vi "Apply Graph Property.vi"(6 "Display State Change Class":T2, 8 "error in (no error)":errorcluster, 9 "Max Range":T1, 10 "XY Graph Property Cluster":T3, 11 "XY Graph":refnum<vi>) -> (0 "error out":errorcluster, 3 "XY Graph":refnum<vi>)   [LabVIEW 2020, in "XY Plot Matrix.lvclass"]
uses:
  <vilib>/Math Plots/2D Math Plots/XY Plot Matrix/XY Plot Matrix/XY Plot Matrix.lvclass
  <vilib>/Math Plots/2D Math Plots/2D Plot/2D Plot/Typedef/Property Cluster.ctl
  <vilib>/Math Plots/2D Math Plots/2D Plot/2D Plot/Typedef/Graph General Property.ctl
  <vilib>/Math Plots/2D Math Plots/2D Plot/2D Plot/Typedef/Scale Array.ctl
  <vilib>/Math Plots/2D Math Plots/2D Plot/2D Plot/Typedef/Scale Cluster.ctl
  <vilib>/Utility/miscctls.llb/LVOffsetAndMultiplierTypeDef.ctl
  <vilib>/Math Plots/2D Math Plots/2D Plot/2D Plot/Typedef/Cursor Property.ctl
  <vilib>/Utility/miscctls.llb/LVCursorListTypeDef.ctl
  <vilib>/Utility/miscctls.llb/LVAnnotationListTypeDef.ctl
  <vilib>/Math Plots/2D Math Plots/2D Plot/Action String/2DMathPlot State Class.ctl
  <vilib>/Math Plots/2D Math Plots/2D Plot/2D Plot/Typedef/Range Cluster.ctl
  <vilib>/Math Plots/2D Math Plots/2D Plot/2D Plot/2D Plot.lvclass
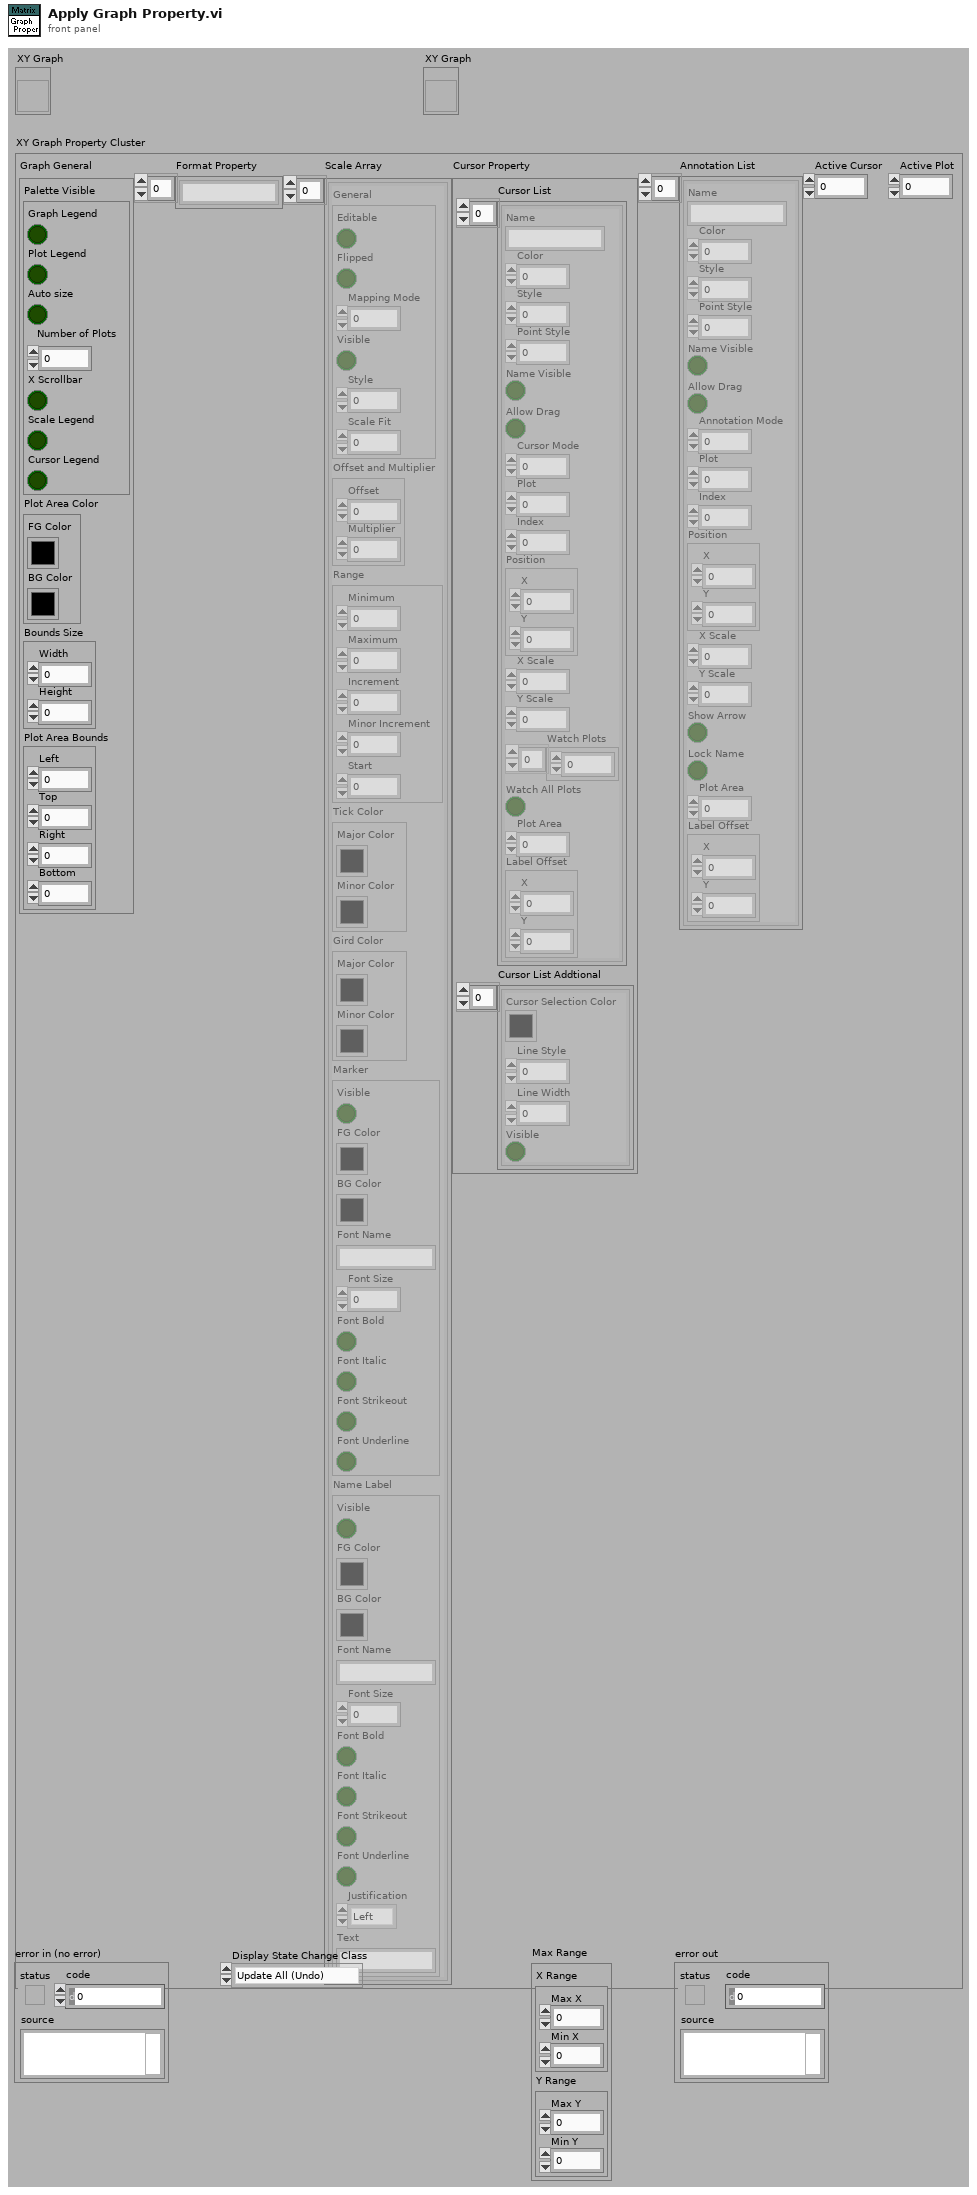
[diagram p1: front panel]
types:
  T1 = typedef "2D Plot.lvclass/Range Cluster.ctl" = cluster{"X Range":cluster{"Max X":dbl, "Min X":dbl}, "Y Range":cluster{"Max Y":dbl, "Min Y":dbl}}
  T2 = typedef "2DMathPlot State Class.ctl" = enum16{"Update All (Undo)", "Update General", "Update Appearance", "Update Format", "Update Scale", "Update Marker", "Update Cursor", "None"}
  T3 = typedef "2D Plot.lvclass/Property Cluster.ctl" = cluster{"Graph General":T4, "Format Property":string[], "Scale Array":T5, "Cursor Property":T8, "Annotation List":T10, "Active Cursor":i32, "Active Plot":i32}
  T4 = typedef "2D Plot.lvclass/Graph General Property.ctl" = cluster{"Palette Visible":cluster{"Graph Legend":bool, "Plot Legend":bool, "Auto size":bool, "Number of Plots":u32, "X Scrollbar":bool, "Scale Legend":bool, "Cursor Legend":bool}, "Plot Area Color":cluster{"FG Color":u32, "BG Color":u32}, "Bounds Size":cluster{"Width":u32, "Height":u32}, "Plot Area Bounds":cluster{"Left":i16, "Top":i16, "Right":i16, "Bottom":i16}}
  T5 = typedef "2D Plot.lvclass/Scale Array.ctl" = T6[]
  T6 = typedef "2D Plot.lvclass/Scale Cluster.ctl" = cluster{"General":cluster{"Editable":bool, "Flipped":bool, "Mapping Mode":u8, "Visible":bool, "Style":u8, "Scale Fit":u8}, "Offset and Multiplier":T7, "Range":cluster{"Minimum":dbl, "Maximum":dbl, "Increment":dbl, "Minor Increment":dbl, "Start":dbl}, "Tick Color":cluster{"Major Color":u32, "Minor Color":u32}, "Gird Color":cluster{"Major Color":u32, "Minor Color":u32}, "Marker":cluster{"Visible":bool, "FG Color":u32, "BG Color":u32, "Font Name":string, "Font Size":u32, "Font Bold":bool, "Font Italic":bool, "Font Strikeout":bool, "Font Underline":bool}, "Name Label":cluster{"Visible":bool, "FG Color":u32, "BG Color":u32, "Font Name":string, "Font Size":u32, "Font Bold":bool, "Font Italic":bool, "Font Strikeout":bool, "Font Underline":bool, "Justification":enum16{"Left", "Center", "Right"}, "Text":string}}
  T7 = typedef "LVOffsetAndMultiplierTypeDef.ctl" = cluster{"Offset":dbl, "Multiplier":dbl}
  T8 = typedef "2D Plot.lvclass/Cursor Property.ctl" = cluster{"Cursor List":T9, "Cursor List Addtional":cluster{"Cursor Selection Color":u32, "Line Style":u8, "Line Width":u8, "Visible":bool}[]}
  T9 = typedef "LVCursorListTypeDef.ctl" = cluster{"Name":string, "Color":u32, "Style":u8, "Point Style":u8, "Name Visible":bool, "Allow Drag":bool, "Cursor Mode":u32, "Plot":i32, "Index":i32, "Position":cluster{"X":dbl, "Y":dbl}, "X Scale":u32, "Y Scale":u32, "Watch Plots":i32[], "Watch All Plots":bool, "Plot Area":i32, "Label Offset":cluster{"X":dbl, "Y":dbl}}[]
  T10 = typedef "LVAnnotationListTypeDef.ctl" = cluster{"Name":string, "Color":u32, "Style":u8, "Point Style":u8, "Name Visible":bool, "Allow Drag":bool, "Annotation Mode":u32, "Plot":i32, "Index":i32, "Position":cluster{"X":dbl, "Y":dbl}, "X Scale":u32, "Y Scale":u32, "Show Arrow":bool, "Lock Name":bool, "Plot Area":i32, "Label Offset":cluster{"X":dbl, "Y":dbl}}[]
  T11 = cluster{"Graph Legend":bool, "Plot Legend":bool, "Auto size":bool, "Number of Plots":u32, "X Scrollbar":bool, "Scale Legend":bool, "Cursor Legend":bool}
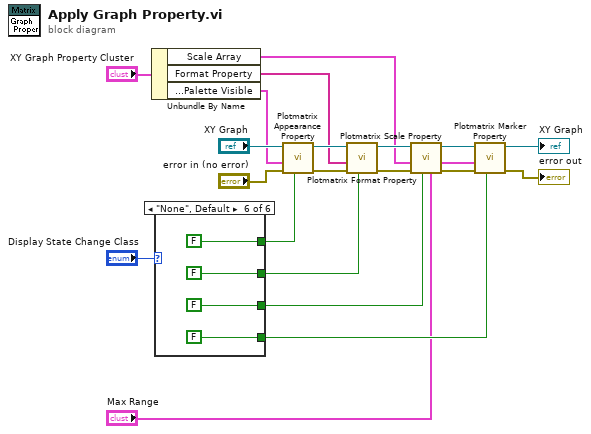
[diagram p0: block diagram]
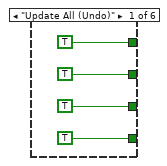
[diagram p2: hidden frame]
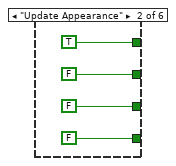
[diagram p3: hidden frame]
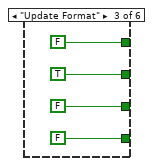
[diagram p4: hidden frame]
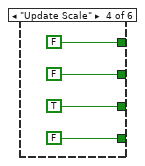
[diagram p5: hidden frame]
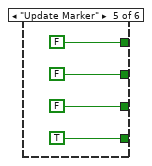
[diagram p6: hidden frame]
diagram:
  n1 = Unbundle By Name("XY Graph Property Cluster") -> ("Scale Array"=w12:T5, "Format Property"=w7:string[], "Graph General.Palette Visible"=w13:T11)
  n2 = case shown="\"None\", Default" "Display State Change Class" {
    tunnel: [TRUE ("Update?") TRUE ("Update?") FALSE ("Update?") FALSE ("Update?") FALSE ("Update?") FALSE ("Update?")] -> w5
    tunnel: [TRUE ("Update?") FALSE ("Update?") TRUE ("Update?") FALSE ("Update?") FALSE ("Update?") FALSE ("Update?")] -> w4
    tunnel: [TRUE ("Update?") FALSE ("Update?") FALSE ("Update?") TRUE ("Update?") FALSE ("Update?") FALSE ("Update?")] -> w3
    tunnel: [TRUE ("Update?") FALSE ("Update?") FALSE ("Update?") FALSE ("Update?") TRUE ("Update?") FALSE ("Update?")] -> w2
    frame "Update All (Undo)" {
    }
    frame "Update Appearance" {
    }
    frame "Update Format" {
    }
    frame "Update Scale" {
    }
    frame "Update Marker" {
    }
    frame "None", Default {
    }
  }
  n3 = call <vilib>:"Plotmatrix Appearance Property.vi"("Update?"=w5, "error in (no error)"="error in (no error)", "Palette Visible"=w13, "Single XY Plot In"="XY Graph") -> ("error out"=w8:errorcluster, "Single XY Plot Out"=w19:refnum<vi>)  [unwired: 1 in, 5 out]
  n4 = call <vilib>:"Plotmatrix Format Property.vi"("Update?"=w4, "error in (no error)"=w8, "Format Property"=w7, "Single XY Plot In"=w19) -> ("error out"=w9:errorcluster, "Single XY Plot Out"=w18:refnum<vi>)  [unwired: 6 out]
  n5 = call <vilib>:"Plotmatrix Scale Property.vi"("Max Range"="Max Range", "Update?"=w3, "error in (no error)"=w9, "Scale Array In"=w12, "Single XY Plot In"=w18) -> ("error out"=w10:errorcluster, "Scale Array Out"=w11:T5, "Single XY Plot Out"=w17:refnum<vi>)  [unwired: 4 out]
  n6 = call <vilib>:"Plotmatrix Marker Property.vi"("Update?"=w2, "error in (no error)"=w10, "Scale Array In"=w11, "Single XY Plot In"=w17) -> ("error out"=→"error out":errorcluster, "Single XY Plot Out"=→"XY Graph":refnum<vi>)  [unwired: 6 out]
